vi "FTW-JSON-Object-GetElement-Bool.vi"(0 "JSON Object":refnum<class "FTW-JSON.lvclass">, 5 "Key":string, 7 "Default Value":bool, 11 "error in":errorcluster) -> (4 "JSON Object out":refnum<class "FTW-JSON.lvclass">, 8 "Value":bool, 10 "Found?":bool, 15 "error out":errorcluster)   [LabVIEW 2014, in "FTW-JSON.lvclass"]
uses:
  FTW-JSON.lvclass
  FTW-JSON.lvclass/FTW-JSON.ctl
  lib/FTW-JSON-Type.ctl
  error/FTW-ERR-ThrowError.vi
  error/FTW-ERR-NoErrorConstant.vi
  error/FTW-ERR-CallChain.vi
  string/FTW-STR-ReplaceWhitespace.vi
panel:
  # "Inputs"
  # "Outputs"
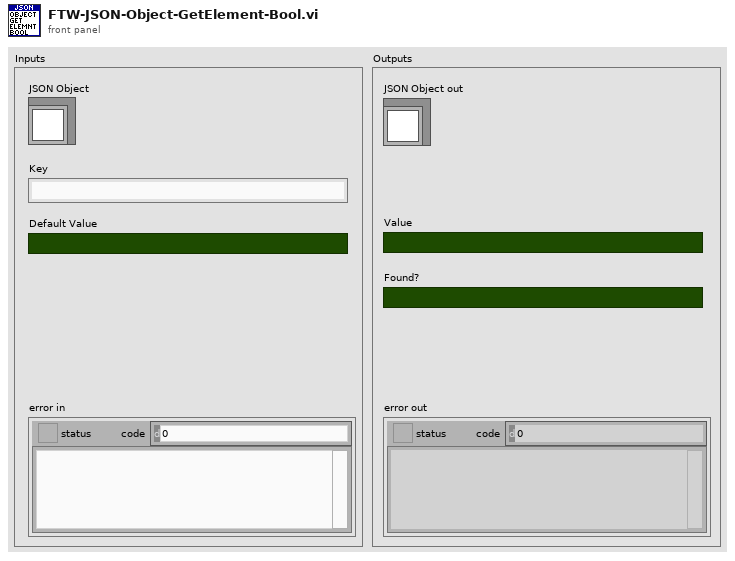
[diagram p1: front panel]
types:
  T1 = typedef "FTW-JSON-Type.ctl" = enum16{"Object", "Array", "String", "Integer", "Floating Point", "true", "false", "null", "undefined"}
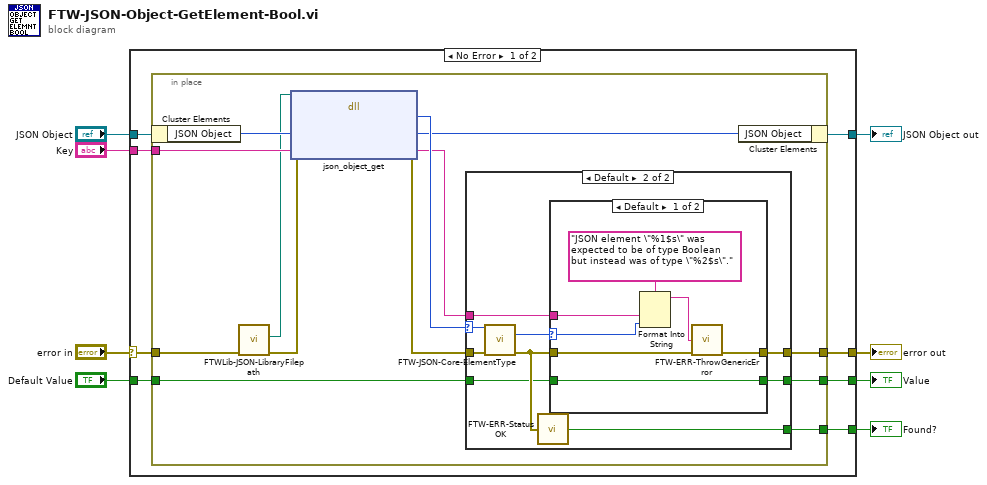
[diagram p0: block diagram]
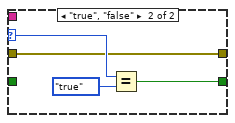
[diagram p3: hidden frame]
diagram:
  n1 = case shown="No Error" "error in" {
    selector: "error in" -> [w16 w54]
    tunnel: [w12 w54] -> w8
    tunnel: [w14 w53] -> w6
    tunnel: "JSON Object" -> [w15 w53]
    tunnel: "Key" -> [w13 _]
    tunnel: [w11 w52] -> w3
    tunnel: [w10 _] -> w2
    tunnel: "Default Value" -> [w9 w52]
    frame No Error {
      n2 = in-place {
        in-place-border: w16 -> [w29]
        in-place-border: w13 -> [w27]
        in-place-border: [w23] -> w12
        in-place-border: [w22] -> w11
        in-place-border: [w19] -> w10
        in-place-border: w9 -> [w17]
        n3 = in-place-cluster #1(w15) -> ("JSON Object"=w28:i64)
        n4 = call "FTWLib-JSON-LibraryFilepath.vi"("error in"=w29) -> ("error out"=w26:errorcluster, "JSON Library Filepath"=w25:path)  [unwired: 9 in]
        n5 = dll-call lib="?" fn="json_object_get"(path in=w25, error in=w26, "JSON Object Pointer"=w28, "Element Key"=w27) -> (error out=w24:errorcluster, "JSON Element Pointer"=w21:i64, "JSON Object Pointer"=w20:i64, "Element Key"=w18:string)  [unwired: 1 in, 1 out]
        n6 = case shown="Default" w21 {
          selector: w21 -> [_ w40]
          tunnel: w24 -> [w31 w36]
          tunnel: [w31 w37] -> w23
          tunnel: [w30 w39] -> w22
          tunnel: [_ w34] -> w19
          tunnel: w18 -> [_ w35]
          tunnel: w17 -> [w30 w32]
          frame 0 {
          }
          frame Default {
            n7 = call "FTW-JSON-Core-ElementType.vi"("JSON Element"=w40, "error in"=w36) -> ("JSON Type"=w38:T1, "error out"=w33:errorcluster)  [unwired: 11 in, 1 out]
            n8 = call "FTW-ERR-StatusOK.vi"("error to check"=w33) -> ("Status OK?"=w34:bool)
            n9 = case shown="Default" w38 {
              selector: w38 -> [w43 w49]
              tunnel: [w41 w50] -> w39
              tunnel: w33 -> [w47 w48]
              tunnel: [w42 w48] -> w37
              tunnel: w35 -> [w44 _]
              tunnel: w32 -> [w41 _]
              frame Default {
                n10 = Format Into String(format string="JSON element \"%1$s\" was expected to be of type Boolean but instead was of type \"%2$s\"." ("Error Message"), w44, w43) -> (resulting string=w45:string)  [unwired: 2 in, 1 out]
                n11 = call "FTW-ERR-ThrowGenericError.vi"("Error Message"=w45, "error in"=w47) -> ("error out"=w42:errorcluster)  [unwired: 13 in]
              }
              frame "true", "false" {
                n12 = Equal?(x=w49, y=FTW-JSON-Type."true" ("x")) -> (x = y?=w50:bool)
              }
            }
          }
        }
        n13 = in-place-cluster #1("JSON Object"=w20) -> (w14:refnum<class "FTW-JSON.lvclass">)
      }
    }
    frame Error {
    }
  }
  "error out" <- w8
  "JSON Object out" <- w6
  "Value" <- w3
  "Found?" <- w2
